vi "Read stored tag set.vi"(8 "error in (no error)":errorcluster, 11 "stored tags":T3[](array[typedef])) -> (0 "error out":errorcluster, 3 "Tags":T1[](array[typedef]))   [LabVIEW 2010, in "Current Value Table.lvlib"]
uses:
  Current Value Table.lvlib
  Type Defs/Tag in Memory.ctl
  Type Defs/Single Tag.ctl
  Type Defs/Data Types.ctl
  Data To ASCII String.vi
  DataTypes/Double_Data To ASCII String.vi
  Read Index.vi
  DataTypes/Double_Read Index.vi
  DataTypes/Array of String_Data To ASCII String.vi
  DataTypes/Array of String_Read Index.vi
  DataTypes/Array of Boolean_Data To ASCII String.vi
  DataTypes/Array of Boolean_Read Index.vi
  DataTypes/Array of Single_Data To ASCII String.vi
  DataTypes/Array of Single_Read Index.vi
  DataTypes/Array of Double_Data To ASCII String.vi
  DataTypes/Array of Double_Read Index.vi
  DataTypes/Array of I8_Data To ASCII String.vi
  DataTypes/Array of I8_Read Index.vi
  DataTypes/Array of I16_Data To ASCII String.vi
  DataTypes/Array of I16_Read Index.vi
  DataTypes/Array of I32_Data To ASCII String.vi
  DataTypes/Array of I32_Read Index.vi
  DataTypes/Array of I64_Data To ASCII String.vi
  DataTypes/Array of I64_Read Index.vi
  DataTypes/Array of U64_Data To ASCII String.vi
  DataTypes/Array of U64_Read Index.vi
  DataTypes/Array of U32_Data To ASCII String.vi
  DataTypes/Array of U32_Read Index.vi
  DataTypes/Array of U16_Data To ASCII String.vi
  DataTypes/Array of U16_Read Index.vi
  DataTypes/Array of U8_Data To ASCII String.vi
  DataTypes/Array of U8_Read Index.vi
  DataTypes/Boolean_Data To ASCII String.vi
  DataTypes/Boolean_Read Index.vi
  DataTypes/String_Data To ASCII String.vi
  DataTypes/String_Read Index.vi
  DataTypes/U8_Data To ASCII String.vi
  DataTypes/U8_Read Index.vi
  DataTypes/U16_Data To ASCII String.vi
  DataTypes/U16_Read Index.vi
  DataTypes/U32_Data To ASCII String.vi
  DataTypes/U32_Read Index.vi
  DataTypes/U64_Data To ASCII String.vi
  DataTypes/U64_Read Index.vi
  DataTypes/I8_Data To ASCII String.vi
  DataTypes/I8_Read Index.vi
  DataTypes/I16_Data To ASCII String.vi
  DataTypes/I16_Read Index.vi
  DataTypes/I32_Data To ASCII String.vi
  DataTypes/I32_Read Index.vi
  DataTypes/I64_Data To ASCII String.vi
  DataTypes/I64_Read Index.vi
  DataTypes/Single_Data To ASCII String.vi
  DataTypes/Single_Read Index.vi
  Memory Block.vi
  DataTypes/Double_Memory Block.vi
  DataTypes/Array of String_Memory Block.vi
  DataTypes/Array of Boolean_Memory Block.vi
  DataTypes/Array of Single_Memory Block.vi
  DataTypes/Array of Double_Memory Block.vi
  DataTypes/Array of I8_Memory Block.vi
  DataTypes/Array of I16_Memory Block.vi
  DataTypes/Array of I32_Memory Block.vi
  DataTypes/Array of I64_Memory Block.vi
  DataTypes/Array of U64_Memory Block.vi
  DataTypes/Array of U32_Memory Block.vi
  DataTypes/Array of U16_Memory Block.vi
  DataTypes/Array of U8_Memory Block.vi
  DataTypes/Boolean_Memory Block.vi
  DataTypes/String_Memory Block.vi
  DataTypes/U8_Memory Block.vi
  DataTypes/U16_Memory Block.vi
  DataTypes/U32_Memory Block.vi
  DataTypes/U64_Memory Block.vi
  DataTypes/I8_Memory Block.vi
  DataTypes/I16_Memory Block.vi
  DataTypes/I32_Memory Block.vi
  DataTypes/I64_Memory Block.vi
  DataTypes/Single_Memory Block.vi
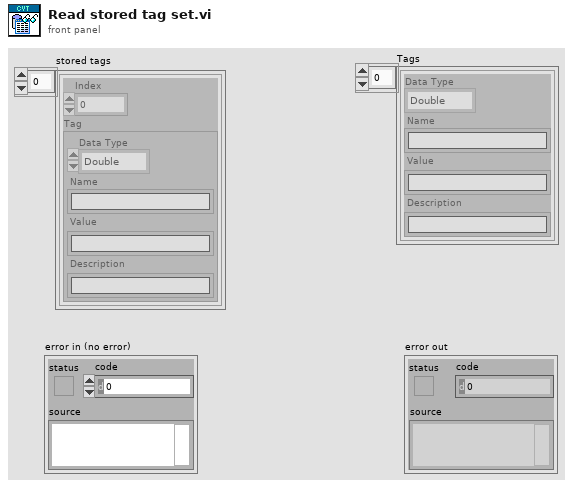
[diagram p1: front panel]
types:
  T1 = typedef "Current Value Table.lvlib/Single Tag.ctl" = cluster{"Data Type":T2, "Name":string, "Value":string, "Description":string}
  T2 = typedef "Current Value Table.lvlib/Data Types.ctl" = enum16{"Double", "Single", "I64", "I32", "I16", "I8", "U64", "U32", "U16", "U8", "String", "Boolean", "Array of U8", "Array of U16", "Array of U32", "Array of U64", "Array of I64", "Array of I32", "Array of I16", "Array of I8", "Array of Double", "Array of Single", "Array of Boolean", "Array of String"}
  T3 = typedef "Current Value Table.lvlib/Tag in Memory.ctl" = cluster{"Index":i32, "Tag":T1}
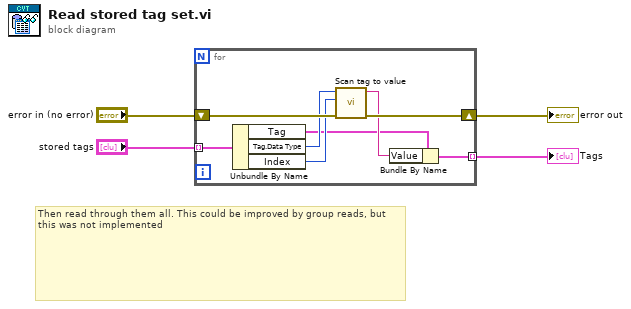
[diagram p0: block diagram]
diagram:
  # "Then read through them all. This could be improved by group reads, but this was not implemented"
  n1 = for {
    shift-right: [w11] -> w2
    shift-left: "error in (no error)" -> [w9]
    tunnel: "stored tags" -> [w12] mode=indexing
    tunnel: [w8] -> w1 mode=indexing
    n2 = Unbundle By Name(w12) -> ("Tag"=w5:T1, "Tag.Data Type"=w7:T2, "Index"=w6:i32)
    n3 = call "Scan tag to value.vi"("error in (no error)"=w9, "Index"=w6, "Data Type"=w7) -> ("error out"=w11:errorcluster, "Value"=w10:string)  [unwired: 7 in]
    n4 = Bundle By Name(cluster=w5, "Value"=w10) -> (w8:T1)
  }
  "error out" <- w2
  "Tags" <- w1
